vi "Convert raw adc to real volts.vi"(6 "Lower resistor (none)":dbl=1.0, 7 "Upper resistor (none)":dbl=1.0, 8 "error in (no error)":errorcluster, 10 "ADC ref (1.6vdc)":dbl=1.6, 11 "Raw ADC value":string) -> (0 "error out":errorcluster, 3 "Real volts":dbl)   [LabVIEW 2013]
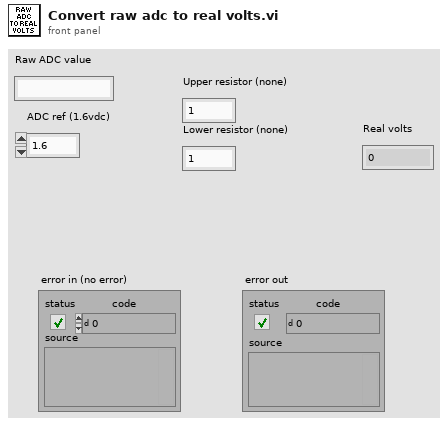
[diagram p1: front panel]
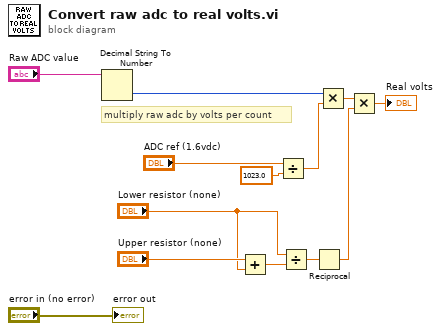
[diagram p0: block diagram]
diagram:
  # "multiply raw adc by volts per count"
  n1 = Decimal String To Number(string="Raw ADC value") -> (number=w12:i32)  [unwired: 2 in, 1 out]
  n2 = Add(x="Upper resistor (none)", y="Lower resistor (none)") -> (x+y=w4:dbl)
  n3 = Divide(x="ADC ref (1.6vdc)", y=1023.0) -> (x/y=w11:dbl)
  n4 = Divide(x="Lower resistor (none)", y=w4) -> (x/y=w2:dbl)
  n5 = Reciprocal(x=w2) -> (1/x=w1:dbl)
  n6 = Multiply(x=w12, y=w11) -> (x*y=w9:dbl)
  n7 = Multiply(x=w9, y=w1) -> (x*y=→"Real volts":dbl)
  "error out" <- "error in (no error)"
